vi "Sum of n Numbers.vi"() -> ()   [LabVIEW 2016]
panel:
  out "Sum":i32
  in  "Sum up till":i32
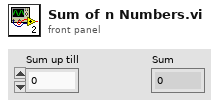
[diagram p1: front panel]
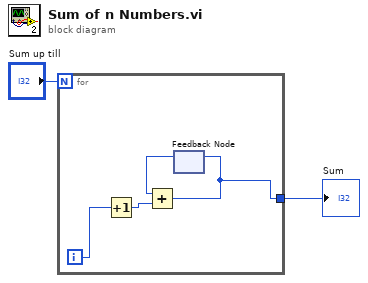
[diagram p0: block diagram]
diagram:
  n1 = for {
    N: "Sum up till" -> [_]
    tunnel: [w3] -> w1
    i -> [w6]
    n2 = Increment(x=w6) -> (x+1=w5:i32)
    n3 = feedback #1() -> (w4:i32)  [unwired: 1 in]
    n4 = Add(x=w4, y=w5) -> (x+y=w3:i32)
    n5 = feedback-in #1(w3) -> ()
  }
  "Sum" <- w1
